vi "Smite All Target.vi"() -> ()   [LabVIEW 2017, in "Bookmark Manager.lvlib" / "Tests.lvlib"]
uses:
  Tests.lvlib
panel:
  in  "Input 3":bool[](array[boolean])=[FALSE, FALSE, FALSE, TRUE, FALSE, FALSE]
  out "Any? 3":bool
  in  "Input 2":bool[](array[boolean])=[FALSE, FALSE, FALSE, TRUE, FALSE, FALSE]
  out "Any? 2":bool
  in  "Input 1":bool[](array[boolean])=[FALSE, FALSE, FALSE, TRUE, FALSE, FALSE]
  out "Any? 1":bool
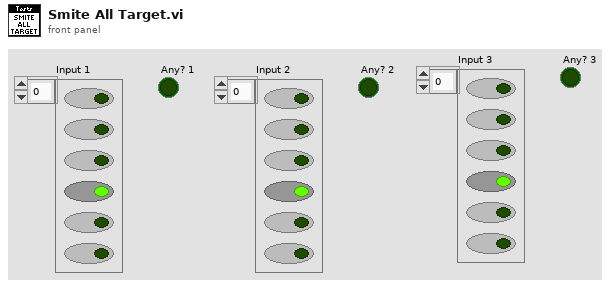
[diagram p1: front panel]
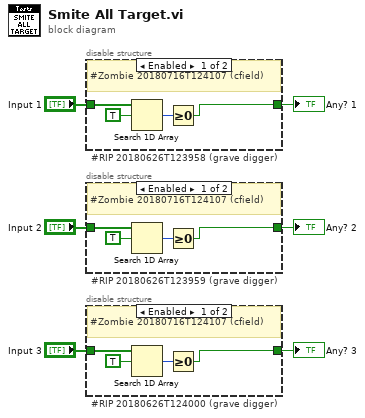
[diagram p0: block diagram]
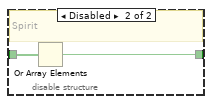
[diagram p2: hidden frame]
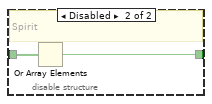
[diagram p3: hidden frame]
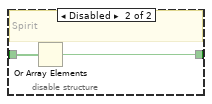
[diagram p4: hidden frame]
diagram:
  n1 = disable-structure "#RIP 20180626T123958 (grave digger)" shown="Enabled" {
    disable-tunnel: "Input 1" -> [w10 w12]
    disable-tunnel: [w9 w11] -> w5
    frame Enabled {
      # "#Zombie 20180716T124107 (cfield)"
      n2 = Search 1D Array(1D array=w10, element=TRUE) -> (index of element=w7:i32)  [unwired: 1 in]
      n3 = Greater Or Equal To 0?(x=w7) -> (x >= 0?=w9:bool)
    }
    frame Disabled {
      # "Spirit"
      n4 = Or Array Elements(Boolean array=w12) -> (logical OR=w11:bool)
    }
  }
  "Any? 1" <- w5
  n5 = disable-structure "#RIP 20180626T123959 (grave digger)" shown="Enabled" {
    disable-tunnel: "Input 2" -> [w16 w18]
    disable-tunnel: [w15 w17] -> w3
    frame Enabled {
      # "#Zombie 20180716T124107 (cfield)"
      n6 = Search 1D Array(1D array=w16, element=TRUE) -> (index of element=w13:i32)  [unwired: 1 in]
      n7 = Greater Or Equal To 0?(x=w13) -> (x >= 0?=w15:bool)
    }
    frame Disabled {
      # "Spirit"
      n8 = Or Array Elements(Boolean array=w18) -> (logical OR=w17:bool)
    }
  }
  "Any? 2" <- w3
  n9 = disable-structure "#RIP 20180626T124000 (grave digger)" shown="Enabled" {
    disable-tunnel: "Input 3" -> [w22 w24]
    disable-tunnel: [w21 w23] -> w1
    frame Enabled {
      # "#Zombie 20180716T124107 (cfield)"
      n10 = Search 1D Array(1D array=w22, element=TRUE) -> (index of element=w19:i32)  [unwired: 1 in]
      n11 = Greater Or Equal To 0?(x=w19) -> (x >= 0?=w21:bool)
    }
    frame Disabled {
      # "Spirit"
      n12 = Or Array Elements(Boolean array=w24) -> (logical OR=w23:bool)
    }
  }
  "Any? 3" <- w1
